vi "Check Chnl Settings.vi"(8 "error in (no error)":errorcluster, 10 "ChnlSettings":T1[](array[typedef]) {"ChnParameter"."Delay (µs)" min=0.0 max=100000000.0 format="%.4f"; "G08_Chnl_Settings"."Pulse Width (µs)" min=0.0 max=8947840.0 format="%#.6f"; "Go and Done Signal"."Done Signal" format="%04x" items=["Local Primary"=1, "Local Secondary"=2, "Local Force"=4, "Master Primary"=16]; "Go and Done Signal"."Go Signal" format="%04x" items=["Local Primary0x1"=1, "Local Secondary0x2"=2, "Local Force 0x4"=4, "Resynchronize 0x8"=8, "Master Prim. 0x10"=16, "Master Sec. 0x20"=32, "Master Force  0x40"=64, "System Clock 0x80"=128, "Delay Clock 0x100"=256, "Inhibit Local 0x200"=512, "Start Local 0x400"=1024, "Start Bus 0x800"=2048, "Step Back Local 0x1000"=4096, "Step Back Bus 0x2000"=8192, "RunCircle 0x4000"=16384, "SyncReload 0x8000"=32768, "From E 0x10000"=65536, "From F 0x20000"=131072, "From Bus 0x40000"=262144]}, 11 "BME_DG_System in":refnum<class "BME_DG_System.lvclass">) -> (0 "error out":errorcluster, 2 "Problem Chnls out":string[](array[string]))   [LabVIEW 2009, in "POLARIS BME DG.lvlib" / "BME_DG_System.lvclass"]
uses:
  BME_DG_System.lvclass
  Chnl Settings Complete.ctl
  LV-BME Interface/ChnlSettings.ctl
  Go_Done_Chnl_Settings.ctl
  GoSignalBits.ctl
  SG08_Chnl_Settings.ctl
  POLARIS BME DG.lvlib
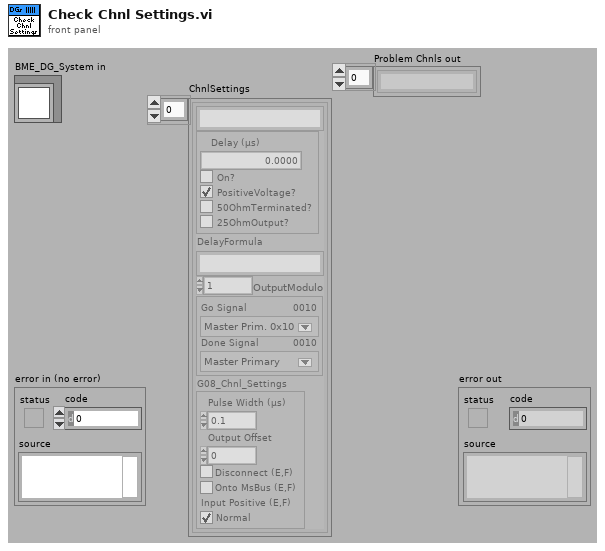
[diagram p1: front panel]
types:
  T1 = typedef "POLARIS BME DG.lvlib/Chnl Settings Complete.ctl" = cluster{"Channel Name":string, "ChnParameter":T2, "DelayFormula":string, "OutputModulo":i32, "Go and Done Signal":T3, "G08_Chnl_Settings":T5}
  T2 = typedef "POLARIS BME DG.lvlib/ChnlSettings.ctl" = cluster{" Delay (µs)":dbl, "On?":bool, "PositiveVoltage?":bool, "50OhmTerminated? ":bool, "25OhmOutput?":bool}
  T3 = typedef "POLARIS BME DG.lvlib/Go_Done_Chnl_Settings.ctl" = cluster{"Go Signal":T4, "Done Signal":u32}
  T4 = typedef "POLARIS BME DG.lvlib/GoSignalBits.ctl" = u32
  T5 = typedef "POLARIS BME DG.lvlib/SG08_Chnl_Settings.ctl" = cluster{"Pulse Width (µs)":dbl, "Output Offset":u32, "Disconnect (E,F)":bool, "Onto MsBus (E,F)":bool, "Input Positive (E,F)":bool}
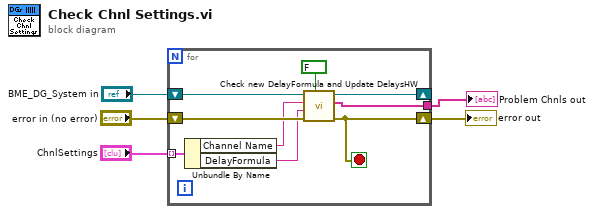
[diagram p0: block diagram]
diagram:
  n1 = for {
    tunnel: "ChnlSettings" -> [w13] mode=indexing
    shift-right: [w7] -> w2
    shift-left: "error in (no error)" -> [w12]
    shift-right: [w8] -> _
    shift-left: "BME_DG_System in" -> [w14]
    tunnel: [w6] -> w1
    stop <- w7 stop-if-true
    n2 = Unbundle By Name(w13) -> ("Channel Name"=w11:string, "DelayFormula"=w10:string)
    n3 = call "Check new DelayFormula and Update DelaysHW.vi"("Update HW?(false)"=FALSE ("Update HW"), "error in (no error)"=w12, "Delay Formula"=w10, "ChnlName"=w11, "BME_DG_System in"=w14) -> ("error out"=w7:errorcluster, "Problem Chnls out"=w6:string[], "BME_DG_System out"=w8:refnum<class "BME_DG_System.lvclass">)  [unwired: 3 in, 1 out]
  }
  "error out" <- w2
  "Problem Chnls out" <- w1
